vi "maszyna stanowa.vi"(8 "Current Time":i32, 9 "Max czas obsługi":dbl, 10 "Queue in":refnum<queue>, 11 "Kasa":T1) -> (2 "Queue in 2":refnum<queue>, 3 "Kasa 2":T1)   [LabVIEW 2014]
doc: "Aktualizuje kasę i kolejkę."
uses:
  Kasy.ctl
  Client.ctl
  LukiBrary.lvlib
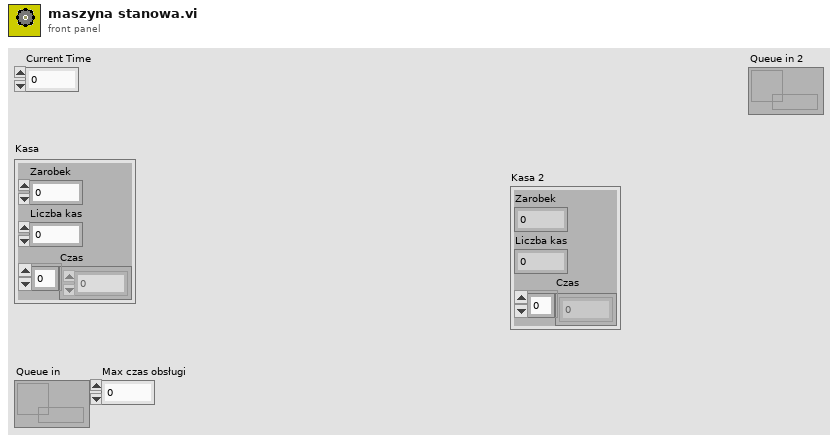
[diagram p1: front panel]
types:
  T1 = typedef "Kasy.ctl" = cluster{"Zarobek":i32, "Liczba kas":u8, "Czas":i32[]}
  T2 = typedef "LukiBrary.lvlib/Client.ctl" = cluster{"Time":i32, "Price":i32}
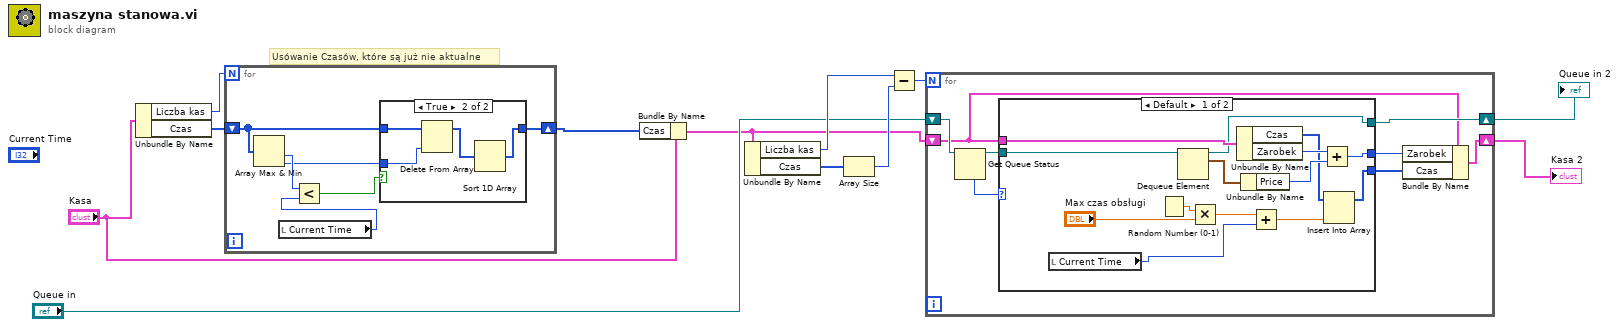
[diagram p0: block diagram]
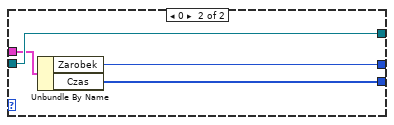
[diagram p2: hidden frame]
diagram:
  # "Usówanie Czasów, które są już nie aktualne"
  n1 = Unbundle By Name("Kasa") -> ("Liczba kas"=w12:u8, "Czas"=w11:i32[])
  n2 = for {
    N: w12 -> [_]
    shift-right: [w14] -> w9
    shift-left: w11 -> [w16]
    n3 = Array Max & Min(array=w16) -> (min value=w18:i32, min index (indices)=w15:i32)  [unwired: 2 out]
    n4 = local read "Current Time"() -> (w13:i32)
    n5 = Less?(x=w18, y=w13) -> (x < y?=w17:bool)
    n6 = case shown="True" w17 {
      tunnel: w16 -> [w19 w23]
      tunnel: w15 -> [_ w22]
      tunnel: [w19 w20] -> w14
      frame False {
      }
      frame True {
        n7 = Delete From Array(array=w23, index=w22) -> (array with subset deleted=w21:i32[])  [unwired: 1 in, 1 out]
        n8 = Sort 1D Array(array=w21) -> (sorted array=w20:i32[])
      }
    }
  }
  n9 = Bundle By Name(cluster="Kasa", "Czas"=w9) -> (w3:T1)
  n10 = Unbundle By Name(w3) -> ("Liczba kas"=w7:u8, "Czas"=w8:i32[])
  n11 = Array Size(array=w8) -> (size(s)=w6:i32)
  n12 = Subtract(x=w7, y=w6) -> (x-y=w5:i32)
  n13 = for {
    N: w5 -> [_]
    shift-right: [w29] -> w1
    shift-left: "Queue in" -> [w31]
    shift-right: [w24] -> w2
    shift-left: w3 -> [w27]
    n14 = Get Queue Status(queue=w31) -> (queue out=w28:refnum<queue>, # elements in queue=w30:i32)  [unwired: 2 in, 6 out]
    n15 = case shown="Default" w30 {
      tunnel: [w43 w49] -> w29
      tunnel: w28 -> [w44 w49]
      tunnel: w27 -> [w45 w48]
      tunnel: [w40 w47] -> w26
      tunnel: [w34 w46] -> w25
      frame Default {
        n16 = local read "Current Time"() -> (w33:i32)
        n17 = Random Number (0-1)() -> (number: 0 to 1=w38:dbl)
        n18 = Dequeue Element(queue=w44) -> (queue out=w43:refnum<queue>, element=w42:T2)  [unwired: 2 in, 2 out]
        n19 = Multiply(x=w38, y="Max czas obsługi") -> (x*y=w36:dbl)
        n20 = Unbundle By Name(w45) -> ("Czas"=w35:i32[], "Zarobek"=w41:i32)
        n21 = Unbundle By Name(w42) -> ("Price"=w39:i32)
        n22 = Add(x=w36, y=w33) -> (x+y=w32:dbl)
        n23 = Add(x=w41, y=w39) -> (x+y=w40:i32)
        n24 = Insert Into Array(array=w35, new element=w32) -> (w34:i32[])  [unwired: 1 in]
      }
      frame 0 {
        n25 = Unbundle By Name(w48) -> ("Zarobek"=w47:i32, "Czas"=w46:i32[])
      }
    }
    n26 = Bundle By Name(cluster=w27, "Zarobek"=w26, "Czas"=w25) -> (w24:T1)
  }
  "Kasa 2" <- w2
  "Queue in 2" <- w1
